vi "FlagStateToColorTest.vi"() -> ()   [LabVIEW 2014]
uses:
  TypeDef/ColorFlags.ctl
  Classes/Flags/ColorEnum.ctl
  Classes/Flags/Flags.lvclass
  Classes/Flags/Flags.lvclass/Flags.ctl
  Classes/Flags/Write State.vi
  Classes/Flags/Write Color.vi
panel:
  in  "Color":T1[](array[typedef])
  in  "State":bool[](array[boolean])
  out "Cluster":T2={"Room Number"=0, "Flag State"=[1, 3, 5, 7]}
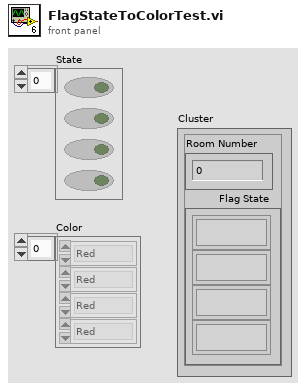
[diagram p1: front panel]
types:
  T1 = typedef "Flags.lvclass/ColorEnum.ctl" = enum8{"Red", "Blue", "Green", "Yellow"}
  T2 = typedef "ColorFlags.ctl" = cluster{"Room Number":u8, "Flag State":u8[]}
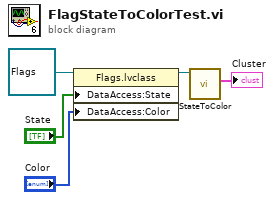
[diagram p0: block diagram]
diagram:
  n1 = property class="Flags.lvclass"(reference=refnum<class "Flags.lvclass"> refnum ("Flags.lvclass"), "DataAccess:State"="State", "DataAccess:Color"="Color") -> (reference out=w4:refnum<class "Flags.lvclass">)  [unwired: 1 in, 1 out]
  n2 = call "StateToColor.vi"("Flags in"=w4) -> ("RoomNumFlags"=→"Cluster":T2)  [unwired: 8 in, 2 out]
